vi "Find String.vi"(8 "error in (no error)":errorcluster caption="错误输入（无错误）", 10 "str":string, 11 "RichText 输入":refnum<class "RichText.lvclass"> caption="DNL_LabVIEW Object in") -> (0 "error out":errorcluster caption="错误输出", 2 "Find":i32, 3 "RichText 输出":refnum<class "RichText.lvclass"> caption="DNL_LabVIEW Object out")   [LabVIEW 2012, in "RichText.lvclass"]
uses:
  RichText.lvclass
  RichText.lvclass/RichText.ctl
  System.Windows.Forms
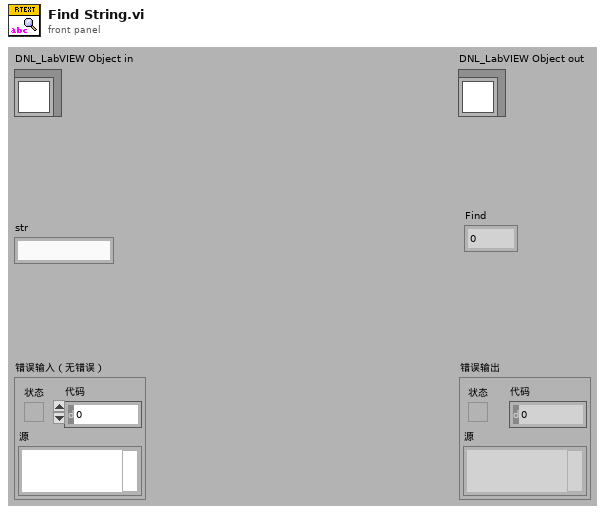
[diagram p1: front panel]
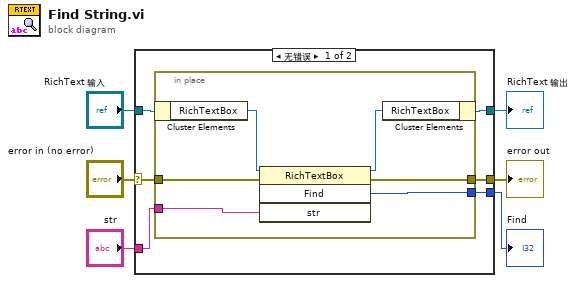
[diagram p0: block diagram]
diagram:
  n1 = case shown="无错误" "error in (no error)" {
    selector: "error in (no error)" -> [w10 w20]
    tunnel: [w9 w20] -> w5
    tunnel: [w8 w19] -> w3
    tunnel: "RichText 输入" -> [w12 w19]
    tunnel: "str" -> [w11 _]
    tunnel: [w7 _] -> w1
    frame No Error {
      n2 = in-place {
        in-place-border: w11 -> [w17]
        in-place-border: w10 -> [w16]
        in-place-border: [w14] -> w9
        in-place-border: [w13] -> w7
        n3 = in-place-cluster #1(w12) -> ("RichTextBox"=w18:refnum<k24>)
        n4 = invoke class="RichTextBox" method="Find"(reference=w18, error in=w16, "str"=w17) -> (reference out=w15:refnum<k24>, error out=w14:errorcluster, "Find"=w13:i32)  [unwired: 1 in, 1 out]
        n5 = in-place-cluster #1("RichTextBox"=w15) -> (w8:refnum<class "RichText.lvclass">)
      }
    }
    frame Error {
    }
  }
  "error out" <- w5
  "RichText 输出" <- w3
  "Find" <- w1
